vi "Swerve Calibrate.vi"(8 "error in (no error)":errorcluster, 11 "Wheel Corner":T1(ring)) -> (0 "error out":errorcluster)   [LabVIEW 2017]
uses:
  <vilib>/Rock Robotics/WPI/ThirdParty/Phoenix-LabVIEW/Motor Controller/Controls/CTRE_Phoenix_MotorControl_ControlMode.ctl
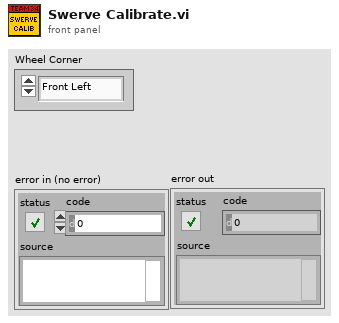
[diagram p1: front panel]
types:
  T1 = enum16{"Front Left", "Front Right", "Back Left", "Back Right"}
  T2 = typedef "CTRE_Phoenix_MotorControl_ControlMode.ctl" = u16
  T3 = typedef "WPI_MotorControlDeviceRef.ctl" = cluster{"DeviceStatus":errorcluster, "Type":T4, "PWM":cluster{"PWM Channel":T5, "DeadBand":T6}, "CAN":cluster{"Device Number":u8, "SetOutput VI Ref":variant, "GetOutput VI Ref":variant, "Enable VI Ref":variant, "Disable VI Ref":variant, "Data":variant}, "Invert":bool, "DIO PWM":cluster{"PWM \"Enable\" Channel":T5, "DIOChannel":T7, "PWM Rate":dbl}}
  T4 = typedef "WPI_MotorControlType.ctl" = enum16{"PWM", "CAN", "DIO PWM"}
  T5 = typedef "FPGA_DIOPWMChannel.ctl" = enum8{"PWM 0", "PWM 1", "PWM 2", "PWM 3", "PWM 4", "PWM 5", "PWM 6", "PWM 7", "PWM 8", "PWM 9", "PWM MXP 0", "PWM MXP 1", "PWM MXP 2", "PWM MXP 3", "PWM MXP 4", "PWM MXP 5", "PWM MXP 6", "PWM MXP 7", "PWM MXP 8", "PWM MXP 9", "Invalid"}
  T6 = typedef "WPI_PWMDeadband.ctl" = cluster{"Name":string, "maxPositivePwm":i32, "minPositivePwm":i32, "centerPwm":i32, "maxNegativePwm":i32, "minNegativePwm":i32, "angularRange":u16}
  T7 = typedef "FPGA_DIOChannel.ctl" = enum8{"DIO 0", "DIO 1", "DIO 2", "DIO 3", "DIO 4", "DIO 5", "DIO 6", "DIO 7", "DIO 8", "DIO 9", "DIO MXP 0", "DIO MXP 1", "DIO MXP 2", "DIO MXP 3", "DIO MXP 4", "DIO MXP 5", "DIO MXP 6", "DIO MXP 7", "DIO MXP 8", "DIO MXP 9", "DIO MXP 10", "DIO MXP 11", "DIO MXP 12", "DIO MXP 13", "DIO MXP 14", "DIO MXP 15", "SPI Port CS1", "SPI Port CS2", "SPI Port CS3", "SPI Port MISO", "SPI Port MOSI", "Invalid"}
  T8 = typedef "WPI_SwitchDevRef.ctl" = cluster{"DevStatus":errorcluster, "DIO Channel":T7, "CntIndex":T9, "Normally Closed":bool}
  T9 = typedef "FPGA_CounterCtrSystemIndex.ctl" = enum8{"Ctr 0", "Ctr 1", "Ctr 2", "Ctr 3", "Ctr 4", "Ctr 5", "Ctr 6", "Ctr 7", "Invalid"}
  T10 = typedef "WPI_EncoderDevRef.ctl" = cluster{"DevStatus":errorcluster, "EncoderIndex":T11, "CounterIndex":T9, "DistancePerCount":dbl, "Decoding Type":T12}
  T11 = typedef "FPGA_EncoderIdx.ctl" = enum8{"Enc 0", "Enc 1", "Enc 2", "Enc 3", "Enc 4", "Enc 5", "Enc 6", "Enc 7", "Invalid"}
  T12 = typedef "WPI_EncoderType.ctl" = enum16{"1x", "2x", "4x"}
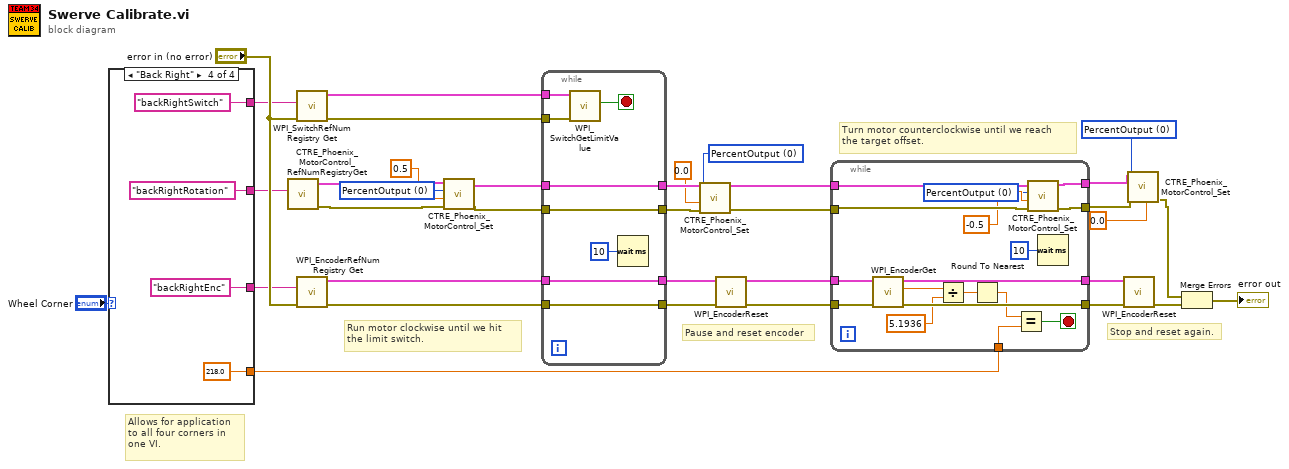
[diagram p0: block diagram]
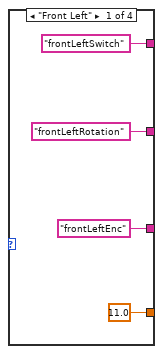
[diagram p2: hidden frame]
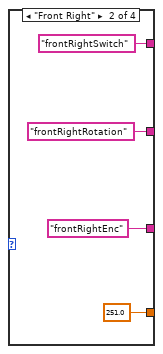
[diagram p3: hidden frame]
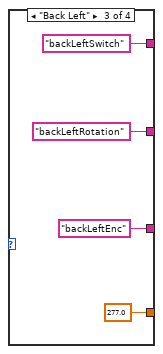
[diagram p4: hidden frame]
diagram:
  w1 = T2 0 items=["PercentOutput"=0, "Position"=1, "Velocity"=2, "Current"=3, "Follower"=5, "MotionProfile"=6, "MotionMagic"=7, "MotionMagicArc"=8, "MotionProfileArc"=10, "Disabled"=15] ("Control Mode")
  w2 = T2 0 items=["PercentOutput"=0, "Position"=1, "Velocity"=2, "Current"=3, "Follower"=5, "MotionProfile"=6, "MotionMagic"=7, "MotionMagicArc"=8, "MotionProfileArc"=10, "Disabled"=15] ("Control Mode")
  w3 = T2 0 items=["PercentOutput"=0, "Position"=1, "Velocity"=2, "Current"=3, "Follower"=5, "MotionProfile"=6, "MotionMagic"=7, "MotionMagicArc"=8, "MotionProfileArc"=10, "Disabled"=15] ("Control Mode")
  # "Allows for application\nto all four corners in \none VI."
  # "Stop and reset again."
  # "Turn motor counterclockwise until we reach\nthe target offset."
  # "Pause and reset encoder"
  # "Run motor clockwise until we hit\nthe limit switch."
  n1 = case shown="\"Back Right\"" "Wheel Corner" {
    tunnel: ["frontLeftSwitch" ("refnum name") "frontRightSwitch" ("refnum name") "backLeftSwitch" ("refnum name") "backRightSwitch" ("refnum name")] -> w21
    tunnel: ["frontLeftRotation" ("refnum name") "frontRightRotation" ("refnum name") "backLeftRotation" ("refnum name") "backRightRotation" ("refnum name")] -> w18
    tunnel: ["frontLeftEnc" ("refnum name") "frontRightEnc" ("refnum name") "backLeftEnc" ("refnum name") "backRightEnc" ("refnum name")] -> w20
    tunnel: [11.0 251.0 277.0 218.0] -> w19
    frame "Front Left" {
    }
    frame "Front Right" {
    }
    frame "Back Left" {
    }
    frame "Back Right" {
    }
  }
  n2 = call <vilib>:"CTRE_Phoenix_MotorControl_RefNumRegistryGet.vi"("refnum name"=w18) -> ("error out"=w17:errorcluster, "PhoenixMotorControlDevRef"=w14:T3)  [unwired: 9 in]
  n3 = call <vilib>:"WPI_SwitchRefNum Registry Get.vi"("error in (no error)"="error in (no error)", "refnum name"=w21) -> ("error out"=w34:errorcluster, "SwitchDevRef"=w35:T8)  [unwired: 8 in]
  n4 = call <vilib>:"WPI_EncoderRefNum Registry Get.vi"("error in (no error)"="error in (no error)", "refnum name"=w20) -> ("error out"=w32:errorcluster, "EncoderDevRef"=w33:T10)  [unwired: 8 in]
  n5 = call <vilib>:"CTRE_Phoenix_MotorControl_Set.vi"("error in (no error)"=w17, "Output"=0.5 ("MotorOutput"), "Control Mode"=w3, "PhoenixMotorControlDevRef"=w14) -> ("error out"=w16:errorcluster, "PhoenixMotorControlDevRef"=w15:T3)  [unwired: 6 in]
  n6 = while {
    tunnel: w16 -> [w56]
    tunnel: w15 -> [w55]
    tunnel: w35 -> [w58]
    tunnel: w34 -> [w59]
    tunnel: [w56] -> w11
    tunnel: [w55] -> w12
    tunnel: [w54] -> w31
    tunnel: w33 -> [w54]
    tunnel: [w53] -> w30
    tunnel: w32 -> [w53]
    stop <- w57 stop-if-true
    n7 = call <vilib>:"WPI_SwitchGetLimitValue.vi"("error in (no error)"=w59, "SwitchDevRef"=w58) -> ("Switch Pressed"=w57:bool)  [unwired: 7 in, 2 out]
    n8 = Wait (ms)(milliseconds to wait=u32 10) -> ()  [unwired: 1 out]
  }
  n9 = call <vilib>:"CTRE_Phoenix_MotorControl_Set.vi"("error in (no error)"=w11, "Output"=0.0, "Control Mode"=w2, "PhoenixMotorControlDevRef"=w12) -> ("error out"=w9:errorcluster, "PhoenixMotorControlDevRef"=w10:T3)  [unwired: 6 in]
  n10 = call <vilib>:"WPI_EncoderReset.vi"("error in (no error)"=w30, "EncoderDevRef"=w31) -> ("error out"=w28:errorcluster, "EncoderDevRef"=w29:T10)  [unwired: 8 in]
  n11 = while {
    tunnel: w29 -> [w76]
    tunnel: w28 -> [w75]
    tunnel: w10 -> [w62]
    tunnel: w9 -> [w65]
    tunnel: [w73] -> w26
    tunnel: [w72] -> w27
    tunnel: [w63] -> w6
    tunnel: [w64] -> w7
    tunnel: w19 -> [w70]
    stop <- w74 stop-if-true
    w60 = T2 0 items=["PercentOutput"=0, "Position"=1, "Velocity"=2, "Current"=3, "Follower"=5, "MotionProfile"=6, "MotionMagic"=7, "MotionMagicArc"=8, "MotionProfileArc"=10, "Disabled"=15] ("Control Mode")
    n12 = call <vilib>:"WPI_EncoderGet.vi"("error in (no error)"=w75, "EncoderDevRef"=w76) -> ("error out"=w73:errorcluster, "Distance"=w68:dbl, "EncoderDevRef"=w72:T10)  [unwired: 4 in, 3 out]
    n13 = Divide(x=w68, y=5.1936) -> (x/y=w67:dbl)
    n14 = Round To Nearest(number=w67) -> (nearest integer value=w71:dbl)
    n15 = Equal?(x=w71, y=w70) -> (x = y?=w74:bool)
    n16 = call <vilib>:"CTRE_Phoenix_MotorControl_Set.vi"("error in (no error)"=w65, "Output"=-0.5, "Control Mode"=w60, "PhoenixMotorControlDevRef"=w62) -> ("error out"=w64:errorcluster, "PhoenixMotorControlDevRef"=w63:T3)  [unwired: 6 in]
    n17 = Wait (ms)(milliseconds to wait=u32 10) -> ()  [unwired: 1 out]
  }
  n18 = call <vilib>:"WPI_EncoderReset.vi"("error in (no error)"=w26, "EncoderDevRef"=w27) -> ("error out"=w24:errorcluster)  [unwired: 8 in, 1 out]
  n19 = call <vilib>:"CTRE_Phoenix_MotorControl_Set.vi"("error in (no error)"=w7, "Output"=0.0, "Control Mode"=w1, "PhoenixMotorControlDevRef"=w6) -> ("error out"=w4:errorcluster)  [unwired: 6 in, 1 out]
  n20 = Merge Errors(w4, w24) -> (→"error out":errorcluster)
